vi "stop-stream_notifier_global.vi"() -> ()   [LabVIEW 2015]
panel:
  in  "stop_stream_notifier":refnum<notifier>
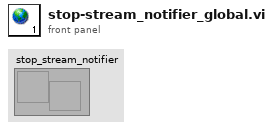
[diagram p1: front panel]
diagram:
